vi "oa_Perform Vectro Average and Weighting.vi"(4 "linear mode":enum16{"One shot", "Auto restart"}(ring), 6 "weighting mode":enum16{"Linear", "Exponential"}(ring)=enum."Exponential", 8 "averages completed":dbl format="%.2f", 9 "number of averages":u32=10 min=1 step=1, 10 "previous array":cdb[](array[numeric]), 11 "Y":cdb[][](array[numeric])) -> (0 "averages completed for buffer":dbl format="%.2f", 1 "average done?":bool, 2 "complex spectrum for buffer":cdb[](array[numeric]), 3 "complex spectrum output":cdb[](array[numeric]), 5 "averages completed for output":dbl format="%.2f")   [LabVIEW 2017, in "SoundVib_Resampling.lvlib"]
uses:
  <vilib>/addons/Sound and Vibration/Order Analysis/Resample Order Tracking/SoundVib_Resampling.lvlib
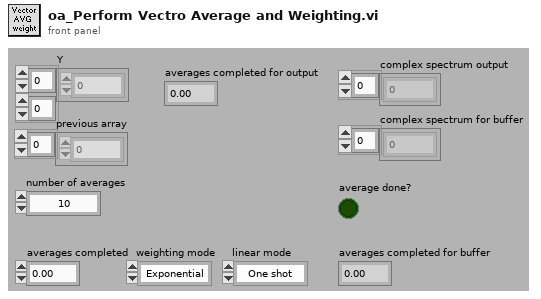
[diagram p1: front panel]
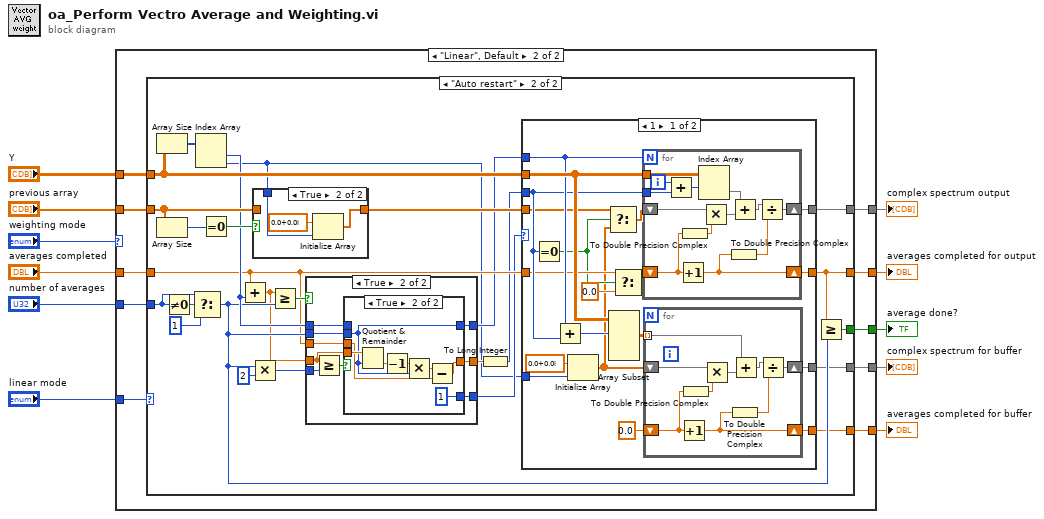
[diagram p0: block diagram]
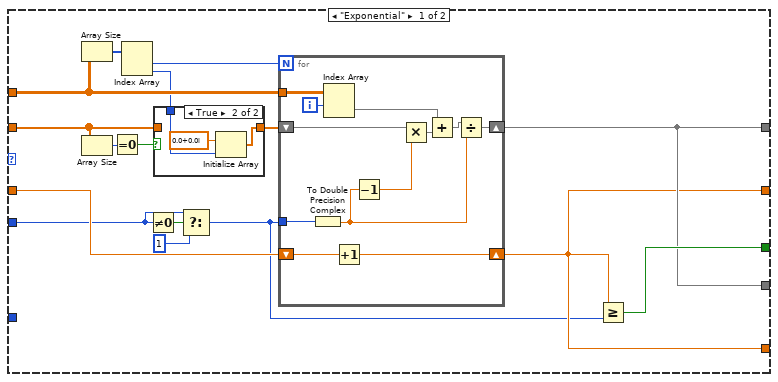
[diagram p2: hidden frame]
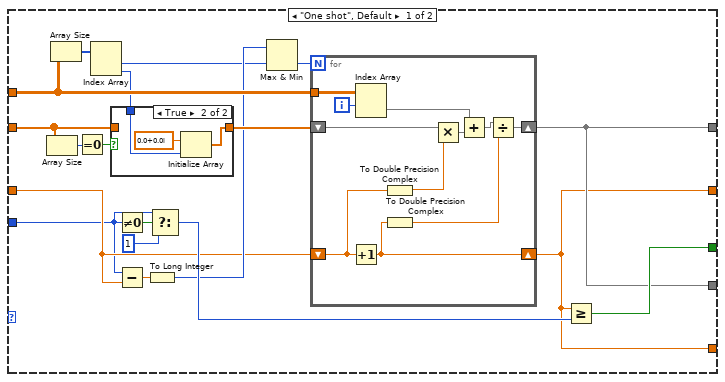
[diagram p4: hidden frame]
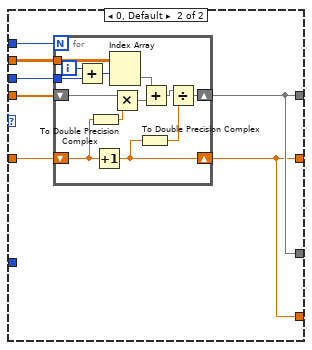
[diagram p6: hidden frame]
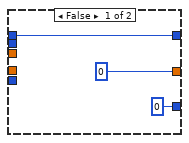
[diagram p7: hidden frame]
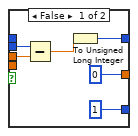
[diagram p8: hidden frame]
diagram:
  n1 = case shown="\"Linear\", Default" "weighting mode" {
    tunnel: [w21 w53] -> w4
    tunnel: "Y" -> [w27 w52]
    tunnel: [w22 w51] -> w5
    tunnel: "previous array" -> [w26 w50]
    tunnel: [w25 w49] -> w1
    tunnel: "averages completed" -> [w24 w48]
    tunnel: "number of averages" -> [w23 w47]
    tunnel: "linear mode" -> [_ w46]
    tunnel: [w22 w45] -> w3
    tunnel: [w21 w44] -> w2
    frame "Exponential" {
      n2 = Array Size(array=w27) -> (size(s)=w20:i32[])
      n3 = Array Size(array=w26) -> (size(s)=w19:i32)
      n4 = Equal To 0?(x=w19) -> (x = 0?=w18:bool)
      n5 = Index Array(array=w20) -> (element #1=w12:i32, element #2=w16:i32)  [unwired: 2 in]
      n6 = Not Equal To 0?(x=w23) -> (x != 0?=w15:bool)
      n7 = case shown="True" w18 {
        tunnel: w26 -> [w28 _]
        tunnel: [w28 w29] -> w17
        tunnel: w16 -> [_ w31]
        frame False {
        }
        frame True {
          n8 = Initialize Array(cdb 0.0+0.0i ("element"), w31) -> (w29:cdb[])
        }
      }
      n9 = Select(t=w23, s=w15, f=u32 1) -> (s? t:f=w13:u32)
      n10 = for {
        N: w12 -> [_]
        tunnel: w27 -> [w36]
        tunnel: w13 -> [w39]
        shift-right: [w37] -> w21
        shift-left: w24 -> [w38]
        shift-right: [w32] -> w22
        shift-left: w17 -> [w33]
        i -> [w34]
        n11 = To Double Precision Complex(1:w39) -> (0:w41:cdb)
        n12 = Index Array(array=w36, index (row)=w34) -> (element=w35:cdb[])  [unwired: 1 in]
        n13 = Increment(x=w38) -> (x+1=w37:dbl)
        n14 = Decrement(x=w41) -> (x-1=w42:cdb)
        n15 = Multiply(x=w33, y=w42) -> (x*y=w40:cdb[])
        n16 = Add(x=w35, y=w40) -> (x+y=w43:cdb[])
        n17 = Divide(x=w43, y=w41) -> (x/y=w32:cdb[])
      }
      n18 = Greater Or Equal?(x=w21, y=w13) -> (x >= y?=w25:bool)
    }
    frame "Linear", Default {
      n19 = case shown="\"Auto restart\"" w46 {
        tunnel: [w55 w90] -> w53
        tunnel: w52 -> [w72 w113]
        tunnel: [w56 w106] -> w51
        tunnel: w50 -> [w68 w109]
        tunnel: [w61 w107] -> w49
        tunnel: w48 -> [w59 w96]
        tunnel: w47 -> [w57 w105]
        tunnel: [w56 w92] -> w45
        tunnel: [w55 w91] -> w44
        frame "One shot", Default {
          n20 = Array Size(array=w68) -> (size(s)=w70:i32)
          n21 = Array Size(array=w72) -> (size(s)=w71:i32[])
          n22 = Equal To 0?(x=w70) -> (x = 0?=w69:bool)
          n23 = Index Array(array=w71) -> (element #1=w58:i32, element #2=w66:i32)  [unwired: 2 in]
          n24 = case shown="True" w69 {
            tunnel: w68 -> [w73 _]
            tunnel: [w73 w74] -> w67
            tunnel: w66 -> [_ w76]
            frame False {
            }
            frame True {
              n25 = Initialize Array(cdb 0.0+0.0i ("element"), w76) -> (w74:cdb[])
            }
          }
          n26 = Not Equal To 0?(x=w57) -> (x != 0?=w65:bool)
          n27 = Subtract(x=w57, y=w59) -> (x-y=w62:dbl)
          n28 = To Long Integer(number=w62) -> (32bit integer=w60:i32)
          n29 = Select(t=w57, s=w65, f=u32 1) -> (s? t:f=w63:u32)
          n30 = Max & Min(x=w60, y=w58) -> (min(x,y)=w54:i32)  [unwired: 1 out]
          n31 = for {
            N: w54 -> [_]
            tunnel: w72 -> [w81]
            shift-right: [w82] -> w55
            shift-left: w59 -> [w83]
            shift-right: [w77] -> w56
            shift-left: w67 -> [w78]
            i -> [w79]
            n32 = Increment(x=w83) -> (x+1=w82:dbl)
            n33 = Index Array(array=w81, index (row)=w79) -> (element=w80:cdb[])  [unwired: 1 in]
            n34 = To Double Precision Complex(1:w83) -> (0:w86:cdb)
            n35 = To Double Precision Complex(1:w82) -> (0:w85:cdb)
            n36 = Multiply(x=w78, y=w86) -> (x*y=w84:cdb[])
            n37 = Add(x=w80, y=w84) -> (x+y=w87:cdb[])
            n38 = Divide(x=w87, y=w85) -> (x/y=w77:cdb[])
          }
          n39 = Greater Or Equal?(x=w55, y=w63) -> (x >= y?=w61:bool)
        }
        frame "Auto restart" {
          n40 = Array Size(array=w113) -> (size(s)=w112:i32[])
          n41 = Array Size(array=w109) -> (size(s)=w111:i32)
          n42 = Not Equal To 0?(x=w105) -> (x != 0?=w104:bool)
          n43 = Select(t=w105, s=w104, f=u32 1) -> (s? t:f=w98:u32)
          n44 = Index Array(array=w112) -> (element #1=w101:i32, element #2=w89:i32)  [unwired: 2 in]
          n45 = Equal To 0?(x=w111) -> (x = 0?=w110:bool)
          n46 = Add(x=w96, y=w101) -> (x+y=w97:dbl)
          n47 = Multiply(x=w98, y=u32 2) -> (x*y=w99:u32)
          n48 = case shown="True" w110 {
            tunnel: w109 -> [w201 _]
            tunnel: [w201 w202] -> w108
            tunnel: w89 -> [_ w204]
            frame False {
            }
            frame True {
              n49 = Initialize Array(cdb 0.0+0.0i ("element"), w204) -> (w202:cdb[])
            }
          }
          n50 = Greater Or Equal?(x=w97, y=w98) -> (x >= y?=w102:bool)
          n51 = case shown="True" w102 {
            tunnel: [w177 w182] -> w95
            tunnel: w101 -> [w177 w180]
            tunnel: [0 w181] -> w94
            tunnel: w97 -> [_ w179]
            tunnel: w99 -> [_ w186]
            tunnel: w98 -> [_ w184]
            tunnel: w96 -> [_ w183]
            tunnel: [0 w178] -> w93
            frame False {
            }
            frame True {
              n52 = Greater Or Equal?(x=w179, y=w186) -> (x >= y?=w185:bool)
              n53 = case shown="True" w185 {
                tunnel: w184 -> [w190 w197]
                tunnel: w183 -> [w192 w194]
                tunnel: [w188 w197] -> w182
                tunnel: [0 w193] -> w181
                tunnel: w180 -> [_ _]
                tunnel: w179 -> [_ w200]
                tunnel: [1 1] -> w178
                frame False {
                  n54 = Subtract(x=w190, y=w192) -> (x-y=w189:dbl)
                  n55 = To Unsigned Long Integer(number=w189) -> (unsigned 32bit integer=w188:u32)
                }
                frame True {
                  n56 = Quotient & Remainder(x=w200, y=w197) -> (floor(x/y)=w199:dbl)  [unwired: 1 out]
                  n57 = Decrement(x=w199) -> (x-1=w198:dbl)
                  n58 = Multiply(x=w198, y=w197) -> (x*y=w195:dbl)
                  n59 = Subtract(x=w195, y=w194) -> (x-y=w193:dbl)
                }
              }
            }
          }
          n60 = To Long Integer(number=w94) -> (32bit integer=w88:i32)
          n61 = case shown="1" w93 {
            tunnel: w113 -> [w127 w161]
            tunnel: w108 -> [w116 w160]
            tunnel: [w132 w156] -> w106
            tunnel: [w131 w155] -> w90
            tunnel: w96 -> [w120 w159]
            tunnel: w95 -> [w125 w158]
            tunnel: w88 -> [w121 w157]
            tunnel: [w129 w156] -> w92
            tunnel: [w130 w155] -> w91
            tunnel: w89 -> [w122 _]
            frame 1 {
              n62 = Equal To 0?(x=w121) -> (x = 0?=w117:bool)
              n63 = Add(x=w125, y=w121) -> (x+y=w126:u32)
              n64 = Initialize Array(cdb 0.0+0.0i ("element"), w122) -> (w114:cdb[])
              n65 = Select(t=w116, s=w117, f=w114) -> (s? t:f=w115:cdb[])
              n66 = Array Subset(array=w127, index (row)=w126) -> (w128:cdb[][])  [unwired: 3 in]
              n67 = Select(t=w120, s=w117, f=0.0) -> (s? t:f=w119:dbl)
              n68 = for {
                N: w125 -> [_]
                tunnel: w127 -> [w149]
                shift-right: [w150] -> w131
                shift-left: w119 -> [w142]
                shift-right: [w146] -> w132
                shift-left: w115 -> [w147]
                tunnel: w121 -> [w143]
                i -> [w144]
                n69 = Add(x=w144, y=w143) -> (x+y=w145:i32)
                n70 = Increment(x=w142) -> (x+1=w150:dbl)
                n71 = To Double Precision Complex(1:w142) -> (0:w153:cdb)
                n72 = Index Array(array=w149, index (row)=w145) -> (element=w148:cdb[])  [unwired: 1 in]
                n73 = Multiply(x=w147, y=w153) -> (x*y=w151:cdb[])
                n74 = To Double Precision Complex(1:w150) -> (0:w152:cdb)
                n75 = Add(x=w148, y=w151) -> (x+y=w154:cdb[])
                n76 = Divide(x=w154, y=w152) -> (x/y=w146:cdb[])
              }
              n77 = for {
                tunnel: w128 -> [w133] mode=indexing
                shift-right: [w136] -> w130
                shift-left: 0.0 -> [w137]
                shift-right: [w134] -> w129
                shift-left: w114 -> [w135]
                n78 = Increment(x=w137) -> (x+1=w136:dbl)
                n79 = To Double Precision Complex(1:w137) -> (0:w140:cdb)
                n80 = Multiply(x=w135, y=w140) -> (x*y=w138:cdb[])
                n81 = To Double Precision Complex(1:w136) -> (0:w139:cdb)
                n82 = Add(x=w133, y=w138) -> (x+y=w141:cdb[])
                n83 = Divide(x=w141, y=w139) -> (x/y=w134:cdb[])
              }
            }
            frame 0, Default {
              n84 = for {
                N: w158 -> [_]
                tunnel: w161 -> [w168]
                shift-right: [w169] -> w155
                shift-left: w159 -> [w170]
                shift-right: [w165] -> w156
                shift-left: w160 -> [w166]
                tunnel: w157 -> [w162]
                i -> [w163]
                n85 = Add(x=w163, y=w162) -> (x+y=w164:i32)
                n86 = To Double Precision Complex(1:w170) -> (0:w173:cdb)
                n87 = Increment(x=w170) -> (x+1=w169:dbl)
                n88 = Index Array(array=w168, index (row)=w164) -> (element=w167:cdb[])  [unwired: 1 in]
                n89 = Multiply(x=w166, y=w173) -> (x*y=w171:cdb[])
                n90 = To Double Precision Complex(1:w169) -> (0:w172:cdb)
                n91 = Add(x=w167, y=w171) -> (x+y=w174:cdb[])
                n92 = Divide(x=w174, y=w172) -> (x/y=w165:cdb[])
              }
            }
          }
          n93 = Greater Or Equal?(x=w90, y=w98) -> (x >= y?=w107:bool)
        }
      }
    }
  }
  "complex spectrum output" <- w5
  "averages completed for buffer" <- w2
  "average done?" <- w1
  "complex spectrum for buffer" <- w3
  "averages completed for output" <- w4
